vi "Clear Arbitrary Waveforms.vi"(8 "error in (no error)":errorcluster, 11 "VISA resource name":refnum<visa-resource-name>="GPIB0::7::INSTR") -> (0 "error out":errorcluster, 3 "VISA resource name dup":refnum<visa-resource-name>)   [LabVIEW 2010]
uses:
  <instrlib>/Agilent 33XXX Series/Agilent 33XXX Series.lvlib
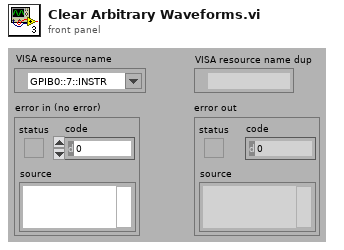
[diagram p1: front panel]
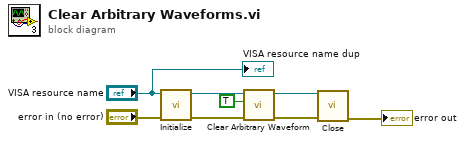
[diagram p0: block diagram]
diagram:
  n1 = call <instrlib>:"Initialize.vi"("error in (no error)"="error in (no error)", "VISA resource name"="VISA resource name") -> ("error out"=w8:errorcluster, "VISA resource name out"=w5:refnum<visa-resource-name>)  [unwired: 8 in]
  n2 = call <instrlib>:"Clear Arbitrary Waveform.vi"("error in (no error)"=w8, "Clear All Waveforms? (F: Disable)"=TRUE, "VISA resource name"=w5) -> ("error out"=w7:errorcluster, "VISA resource name out"=w6:refnum<visa-resource-name>)  [unwired: 7 in]
  n3 = call <instrlib>:"Close.vi"("error in (no error)"=w7, "VISA resource name"=w6) -> ("error out"=→"error out":errorcluster)  [unwired: 9 in]
  "VISA resource name dup" <- "VISA resource name"
